vi "Msg.vi"(7 "jettl in":refnum<class "jettl.lvclass">, 11 "Last Ack Created Event Msg Strategy in":refnum<class "Last Ack Created Event Msg Strategy.lvclass">) -> (5 "jettl out":refnum<class "jettl.lvclass">)   [LabVIEW 2021, in "jettl.lvlib" / "Last Ack Created Event Msg Strategy.lvlib" / "Last Ack Created Event Msg Strategy.lvclass"]
uses:
  Last Ack Created Event Msg Strategy.lvclass
  jettl/jettl.lvclass
  jettl Msg Last Ack Created Event/jettl Msg Last Ack Created Event.lvclass
  Last Ack Created Event Msg Strategy.lvclass/Last Ack Created Event Msg Strategy.ctl
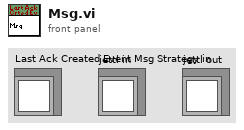
[diagram p1: front panel]
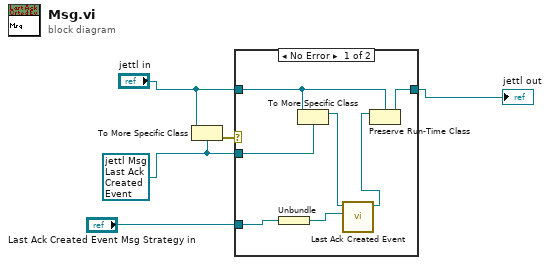
[diagram p0: block diagram]
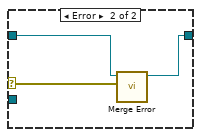
[diagram p2: hidden frame]
diagram:
  w3 = refnum<class "jettl Msg Last Ack Created Event.lvclass"> refnum ("Event Last Ack.lvlib:Event Last Ack.lvclass")
  n1 = To More Specific Class(target class=w3, reference="jettl in") -> (error out=w5:errorcluster)  [unwired: 1 in, 1 out]
  n2 = case shown="No Error" w5 {
    selector: w5 -> [_ w15]
    tunnel: [w10 w13] -> w1
    tunnel: "jettl in" -> [w11 w14]
    tunnel: w3 -> [w12 _]
    tunnel: "Last Ack Created Event Msg Strategy in" -> [w7 _]
    frame No Error {
      n3 = Unbundle(w7) -> (w6:refnum<class "Event.lvclass">)
      n4 = To More Specific Class(target class=w12, reference=w11) -> (specific class reference=w9:refnum<class "jettl Msg Last Ack Created Event.lvclass">)  [unwired: 1 in, 1 out]
      n5 = call-dynamic "Last Ack Created Event.vi"("Event"=w6, "jettl Msg Last Ack Created Event in"=w9) -> ("jettl Msg Last Ack Created Event out"=w8:refnum<class "jettl Msg Last Ack Created Event.lvclass">)  [unwired: 9 in]
      n6 = Preserve Run-Time Class(object in=w8, 2:w11) -> (object out=w10:refnum<class "jettl.lvclass">)  [unwired: 1 in, 1 out]
    }
    frame Error {
      n7 = call-dynamic "Merge Error.vi"("Error"=w15, "jettl Msg Merge Error in"=w14) -> ("jettl Msg Merge Error out"=w13:refnum<class "jettl.lvclass">)  [unwired: 9 in]
    }
  }
  "jettl out" <- w1
